vi "AlliGator Sliced Analysis Initialization.vi"(8 "Iteration (0)":i32, 10 "Slices Definition":T1 {"# Replicas" min=1; "# Elements" min=0; "Min # Data Points/Slice" min=1; "Lower Percentile" min=0.0 max=100.0; "Upper Percentile" min=0.0 max=100.0; "Step Size" min=0.0; "# Steps" min=1}, 11 "tau(I) Plot":cluster{"X Array":dbl[], "Y Array":dbl[]}) -> (0 "[delta I_i]":dbl[](array[numeric]), 1 "[I_i]":dbl[](array[numeric]), 2 "[tau]":dbl[](array[numeric]), 3 "Sorted [I]":dbl[](array[numeric]), 4 "Valid Slices?":bool)   [LabVIEW 2021, in "AlliGator Lifetime & Other Parameters.lvlib"]
uses:
  AlliGator Lifetime & Other Parameters.lvlib
  Graphs/XY Graph/XY Graph Sliced Mean & SDV Step Definition.ctl
  AlliGator Intensity Slice Definition.ctl
  Graphs/XY Graph/XY Graph Sliced CV Abscissa Location.ctl
  Arrays/Linear Ramp End Options.ctl
  00e66e01-47b8-4b11-9c79-51fb075d7779.vi
  <userlib>/_OpenG.lib/array/array.llb/Sort 1D Array (DBL)__ogtk.vi
  <userlib>/_OpenG.lib/array/array.llb/Reorder 1D Array2 (DBL)__ogtk.vi
  Arrays/Arrays.lvlib
  Comparison/Comparison.lvlib
  <userlib>/_OpenG.lib/array/array.llb/openg_array.lvlib
  Graphs/XY Graph/XY Graph Add-Ons.lvlib
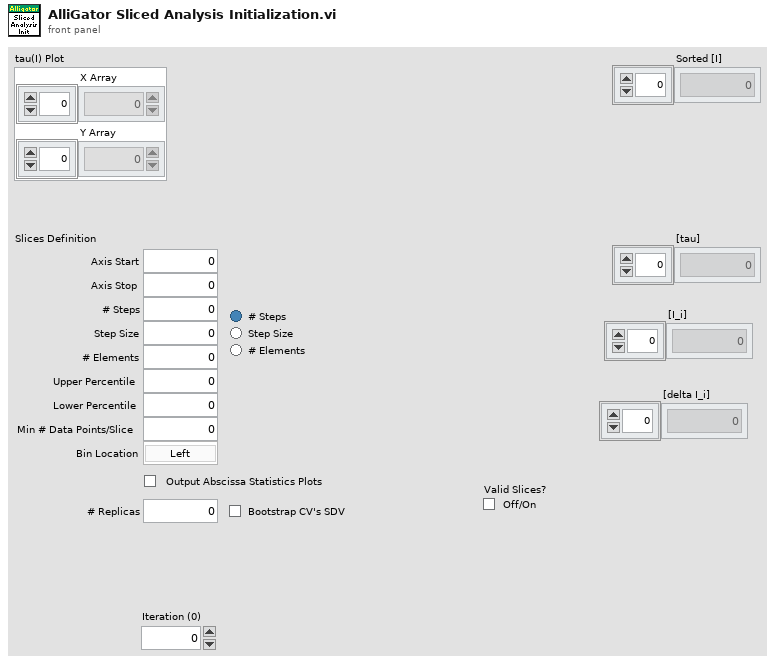
[diagram p1: front panel]
types:
  T1 = typedef "XY Graph Add-Ons.lvlib/XY Graph Sliced Mean & SDV Step Definition.ctl" = cluster{"Axis Start":dbl, "Axis Stop":dbl, "# Steps":i32, "Step Size":dbl, "Step Definition":T2, "Upper Percentile":dbl, "Lower Percentile":dbl, "Min # Data Points/Slice":i32, "Output Abscissa Statistics Plots":bool, "Bin Location":T3, "# Elements":i32, "Bootstrap CV's SDV":bool, "# Replicas":i32}
  T2 = typedef "AlliGator Lifetime & Other Parameters.lvlib/AlliGator Intensity Slice Definition.ctl" = enum32{"# Steps", "Step Size", "# Elements"}
  T3 = typedef "XY Graph Add-Ons.lvlib/XY Graph Sliced CV Abscissa Location.ctl" = enum16{"Left", "Center", "Mean", "Right"}
  T4 = typedef "Arrays.lvlib/Linear Ramp End Options.ctl" = enum16{"Include Min/Exclude Max", "Exclude Min/Include Max", "Include Both Ends", "Exclude Both Ends"}
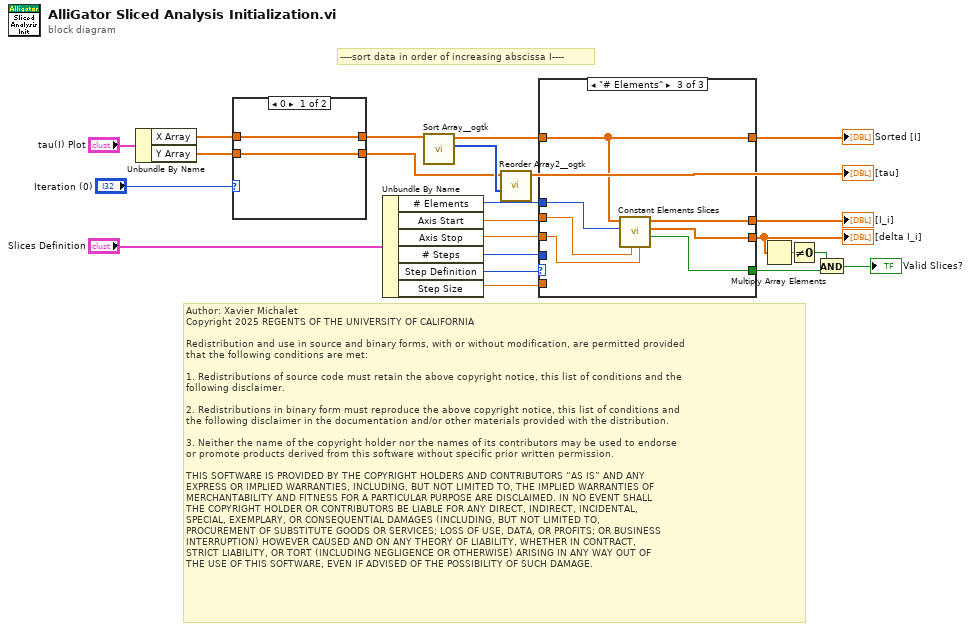
[diagram p0: block diagram]
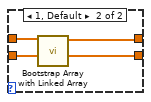
[diagram p2: hidden frame]
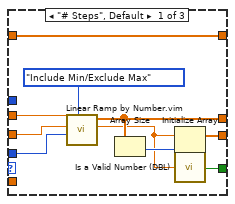
[diagram p3: hidden frame]
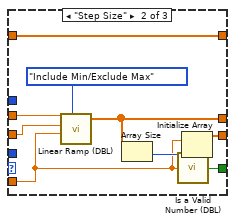
[diagram p4: hidden frame]
diagram:
  # "Author: Xavier Michalet\nCopyright 2025 REGENTS OF THE UNIVERSITY OF CALIFORNIA\n\nRedistribution and use in source and binary forms, with or without modification, are permitted provided\nthat the following conditions are met:\n\n1. Redistributions of source code must retain the above copyright notice, this list of conditions and the\nfollowing disclaimer.\n\n2. Redistributions in binary form must reproduce the above copyright notice, this list of conditions and\nthe following disclaimer in the documentation and/or other materials provided with the distribution.\n\n3. Neither the name of the copyright holder nor the names of its contributors may be used to endorse \nor promote products derived from this software without specific prior written permission.\n\nTHIS SOFTWARE IS PROVIDED BY THE COPYRIGHT HOLDERS AND CONTRIBUTORS “AS IS” AND ANY \nEXPRESS OR IMPLIED WARRANTIES, INCLUDING, BUT NOT LIMITED TO, THE IMPLIED WARRANTIES OF\nMERCHANTABILITY AND FITNESS FOR A PARTICULAR PURPOSE ARE DISCLAIMED. IN NO EVENT SHALL\nTHE COPYRIGHT HOLDER OR CONTRIBUTORS BE LIABLE FOR ANY DIRECT, INDIRECT, INCIDENTAL, \nSPECIAL, EXEMPLARY, OR CONSEQUENTIAL DAMAGES (INCLUDING, BUT NOT LIMITED TO, \nPROCUREMENT OF SUBSTITUTE GOODS OR SERVICES; LOSS OF USE, DATA, OR PROFITS; OR BUSINESS\nINTERRUPTION) HOWEVER CAUSED AND ON ANY THEORY OF LIABILITY, WHETHER IN CONTRACT, \nSTRICT LIABILITY, OR TORT (INCLUDING NEGLIGENCE OR OTHERWISE) ARISING IN ANY WAY OUT OF\nTHE USE OF THIS SOFTWARE, EVEN IF ADVISED OF THE POSSIBILITY OF SUCH DAMAGE."
  # "----sort data in order of increasing abscissa I----"
  n1 = Unbundle By Name("tau(I) Plot") -> ("X Array"=w4:dbl[], "Y Array"=w2:dbl[])
  n2 = case shown="0" "Iteration (0)" {
    tunnel: w4 -> [w25 w29]
    tunnel: [w25 w27] -> w3
    tunnel: w2 -> [w24 w28]
    tunnel: [w24 w26] -> w1
    frame 0 {
    }
    frame 1, Default {
      n3 = call "Bootstrap Array with Linked Array.vi"("Linked Array in"=w28, "Array in"=w29) -> ("Linked Array out"=w26:dbl[], "Bootstrapped Array"=w27:dbl[])  [unwired: 8 in]
    }
  }
  n4 = Unbundle By Name("Slices Definition") -> ("# Elements"=w18:i32, "Axis Start"=w19:dbl, "Axis Stop"=w20:dbl, "# Steps"=w21:i32, "Step Definition"=w22:T2, "Step Size"=w23:dbl)
  n5 = call-poly <userlib>:"Sort Array__ogtk.vi"("Array in"=w3) -> ("Sorted Pointers"=w7:i32[], "Sorted Array out"=w13:dbl[])  [unwired: 9 in]
  n6 = call-poly <userlib>:"Reorder Array2__ogtk.vi"("indices"=w7, "array"=w1) -> ("reordered array"=→"[tau]":dbl[])  [unwired: 9 in]
  n7 = case shown="\"# Elements\"" w22 {
    tunnel: w19 -> [w39 w48 w50]
    tunnel: w20 -> [w38 w47 w51]
    tunnel: w21 -> [w37 _ _]
    tunnel: [w34 w42 w53] -> w10
    tunnel: [w33 w43 w54] -> w9
    tunnel: w23 -> [_ w40 _]
    tunnel: w13 -> [w35 w45 w55]
    tunnel: [w35 w45 w55] -> w14
    tunnel: w18 -> [_ _ w49]
    tunnel: [w31 w41 w52] -> w15
    frame "# Steps", Default {
      n8 = call "Linear Ramp by Number.vim"("Options"=Linear_Ramp_End_Options."Include Min/Exclude Max", "# Steps (1)"=w37, "End (1)"=w38, "Start (0)"=w39) -> ("Step Size"=w30:dbl, "Ramp"=w33:dbl[])  [unwired: 5 in, 1 out]
      n9 = Array Size(array=w33) -> (size(s)=w32:i32)
      n10 = Initialize Array(w30, w32) -> (w34:dbl[])
      n11 = call "Is a Valid Number (DBL).vi"("Number"=w30) -> ("Valid Number?"=w31:bool)  [unwired: 8 in]
    }
    frame "Step Size" {
      n12 = call "Linear Ramp (DBL).vi"("Options"=Linear_Ramp_End_Options."Include Min/Exclude Max", "Delta"=w40, "Max"=w47, "Min"=w48) -> ("Ramp"=w43:dbl[])  [unwired: 5 in, 2 out]
      n13 = Array Size(array=w43) -> (size(s)=w44:i32)
      n14 = call "Is a Valid Number (DBL).vi"("Number"=w40) -> ("Valid Number?"=w41:bool)  [unwired: 8 in]
      n15 = Initialize Array(w40, w44) -> (w42:dbl[])
    }
    frame "# Elements" {
      n16 = call "Constant Elements Slices.vi"("Array Stop (NaN: last)"=w51, "Array Start (NaN: first)"=w50, "# Elements"=w49, "Sorted Array in"=w55) -> ("Valid Number?"=w52:bool, "Bin Widths"=w53:dbl[], "Bin Bounds"=w54:dbl[])  [unwired: 4 in, 1 out]
    }
  }
  "Sorted [I]" <- w14
  "[delta I_i]" <- w10
  "[I_i]" <- w9
  n17 = Multiply Array Elements(1:w10) -> (0:w16:dbl)
  n18 = Not Equal To 0?(x=w16) -> (x != 0?=w11:bool)
  n19 = And(x=w11, y=w15) -> (x .and. y?=→"Valid Slices?":bool)
